vi "Read Child Position.vi"(8 "error in (no error)":errorcluster, 11 "MDI serialize in":refnum<class "MDI serialize.lvclass">) -> (0 "error out":errorcluster, 2 "Position":T1, 3 "MDI serialize out":refnum<class "MDI serialize.lvclass">)   [LabVIEW 2016, in "MDI serialize.lvclass"]
uses:
  MDI serialize.lvclass
  protected/Postion.ctl
  MDI serialize.lvclass/MDI serialize.ctl
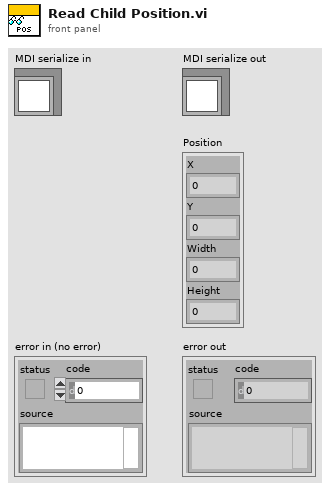
[diagram p1: front panel]
types:
  T1 = typedef "Postion.ctl" = cluster{"X":i32, "Y":i32, "Width":i32, "Height":i32}
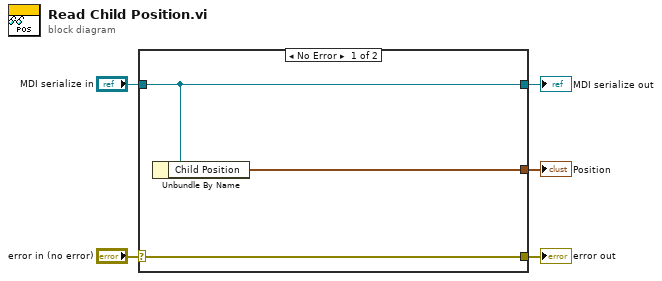
[diagram p0: block diagram]
diagram:
  n1 = case shown="No Error" "error in (no error)" {
    selector: "error in (no error)" -> [w8 w9]
    tunnel: [w8 w9] -> w4
    tunnel: [w7 w10] -> w2
    tunnel: "MDI serialize in" -> [w7 w10]
    tunnel: [w6 _] -> w1
    frame No Error {
      n2 = Unbundle By Name(w7) -> ("Child Position"=w6:T1)
    }
    frame Error {
    }
  }
  "error out" <- w4
  "MDI serialize out" <- w2
  "Position" <- w1
